vi "FrontPanel.vi"() -> ()   [LabVIEW 2017, in "WaveformGenerator.lvlib"]
uses:
  WaveformGenerator.lvlib
  WaveformSpecs.ctl
  WaveformGeneratorInterfaceRef.ctl
  <vilib>/DAQmx/write.llb/DAQmx Write (Analog 1D Wfm NChan NSamp).vi
  MessageQueue/QueueOperations/Enqueue Message (Single).vi
  FrontPanelReferences.vi
  <vilib>/DAQmx/miscellaneous.llb/DAQmx Fill In Error Info.vi
  MessageQueue/MessageQueue.lvlib
panel:
  in  "Field^2":dbl step=0.25
  in  "Waveform Specification":T1
  in  "Enum":enum16{"Initialize", "Idle", "Log", "Stop"}(ring)
  in  "Freq":dbl
  in  "Cone":bool
  in  "Radius":dbl step=0.025
  in  "Angle":dbl
  in  "stop":bool
  in  "OUT":bool caption="ON/OFF"
  out "Waveform Graph":waveform(dbl)[](graph)
  in  "Waveform Z":string(combo)="0" caption="Waveform"
  in  "Offset Z":dbl caption="Offset" min=-10.0 max=10.0 step=0.1
  in  "Phase Z":dbl caption="Phase" min=0.0 max=360.0 step=1.0
  in  "Amplitude Z":dbl caption="Amplitude" min=0.0 max=10.0 step=0.1
  in  "Frequency Z":dbl caption="Frequency" min=0.0 max=1000.0 step=0.1
  in  "Waveform Y":string(combo)="0" caption="Waveform"
  in  "Offset Y":dbl caption="Offset" min=-10.0 max=10.0 step=0.1
  in  "Phase Y":dbl caption="Phase" min=0.0 max=360.0 step=1.0
  in  "Amplitude Y":dbl caption="Amplitude" min=0.0 max=10.0 step=0.1
  in  "Frequency Y":dbl caption="Frequency" min=0.0 max=1000.0 step=0.1
  in  "Waveform X":string(combo)="0" caption="Waveform"
  in  "Offset X":dbl caption="Offset" min=-10.0 max=10.0 step=0.1
  in  "Phase X":dbl caption="Phase" min=0.0 max=360.0 step=1.0
  in  "Amplitude X":dbl caption="Amplitude" min=0.0 max=10.0 step=0.1
  in  "Frequency X":dbl caption="Frequency" min=0.0 max=1000.0 step=0.1
  # "Z Axis Coil"
  # "Y Axis Coil"
  # "X Axis Coil"
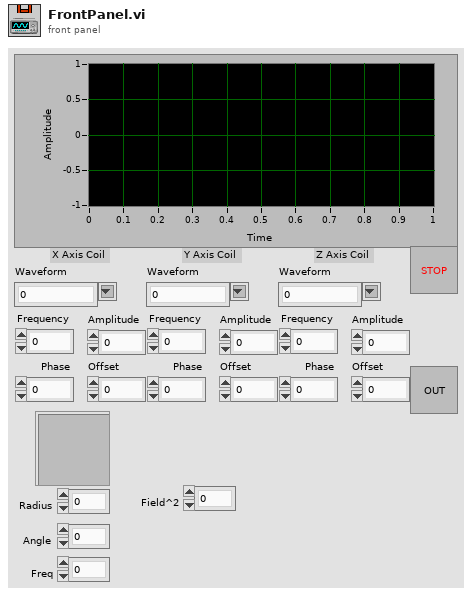
[diagram p1: front panel]
types:
  T1 = typedef "WaveformGenerator.lvlib/WaveformSpecs.ctl" = cluster{"X SignalType":enum16{"Sine Wave", "Triangle Wave", "Square Wave", "Sawtooth Wave"}, "X Offset":dbl, "X Frequency":dbl, "X Amplitude":dbl, "X Phase":dbl, "Y SignalType":enum16{"Sine Wave", "Triangle Wave", "Square Wave", "Sawtooth Wave"}, "Y Offset":dbl, "Y Frequency":dbl, "Y Amplitude":dbl, "Y Phase":dbl, "Z SignalType":enum16{"Sine Wave", "Triangle Wave", "Square Wave", "Sawtooth Wave"}, "Z Offset":dbl, "Z Frequency":dbl, "Z Amplitude":dbl, "Z Phase":dbl}
  T2 = typedef "WaveformGenerator.lvlib/WaveformGeneratorInterfaceRef.ctl" = cluster{"Waveform X":refnum<vi>, "Waveform Y":refnum<vi>, "Waveform Z":refnum<vi>, "Amplitude X":refnum<vi>, "Amplitude Y":refnum<vi>, "Amplitude Z":refnum<vi>, "Frequency X":refnum<vi>, "Frequency Y":refnum<vi>, "Frequency Z":refnum<vi>, "Phase X":refnum<vi>, "Phase Y":refnum<vi>, "Phase Z":refnum<vi>, "Offset X":refnum<vi>, "Offset Y":refnum<vi>, "Offset Z":refnum<vi>, "Stop":refnum<vi>, "On/Off":refnum<vi>, "Field^2":refnum<vi>}
  T3 = typedef "WaveformGenerator.lvlib/MessageQueue.lvlib/All Message Queues.ctl" = cluster{" Interface":refnum<queue>, "Log":refnum<queue>}
  T4 = cluster{"seconds since 1Jan1904":timestamp, "Waveform Specification":T1}
  T5 = enum16{"open", "replace", "create", "open or create", "replace or create", "replace or create with confirmation"}
  T6 = cluster{"Cone":bool, "Angle":dbl, "Radius":dbl, "Freq":dbl}
  T7 = cluster{"seconds since 1Jan1904":timestamp, "Waveform Specification out":T1}
  T8 = enum16{"Sine Wave", "Triangle Wave", "Square Wave", "Sawtooth Wave"}
  T9 = cluster{"Cone":bool, "Angle":dbl, dbl, "Freq":dbl}
  T10 = cluster{"Waveform Specification":T1, "NewVal":bool}
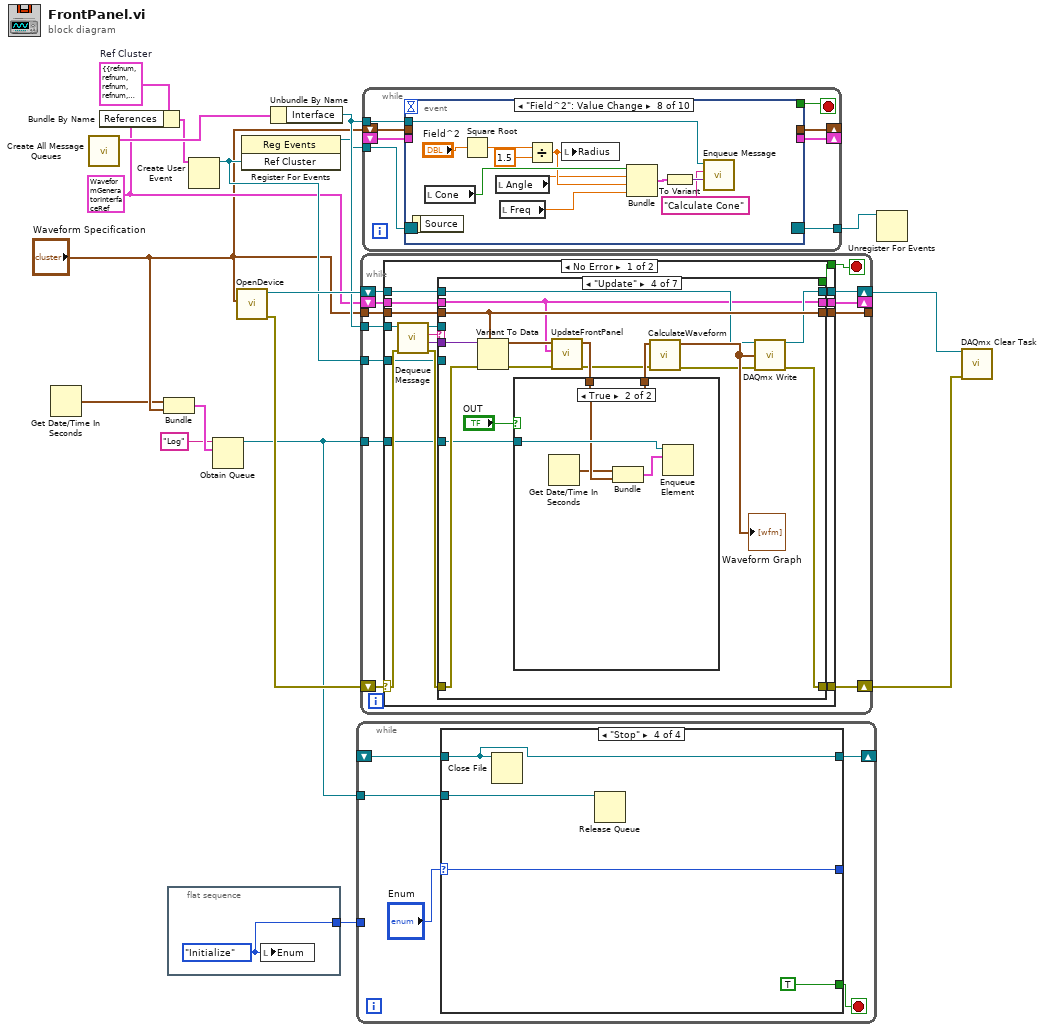
[diagram p0: block diagram]
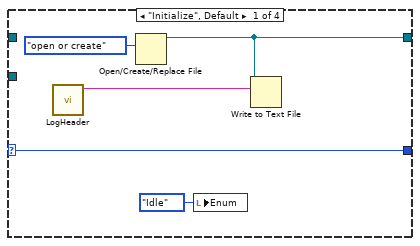
[diagram p2: hidden frame]
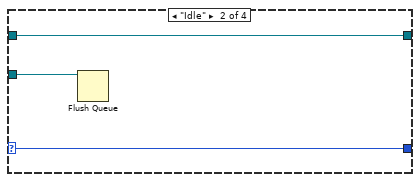
[diagram p3: hidden frame]
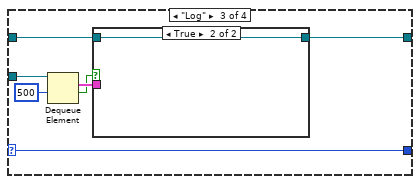
[diagram p4: hidden frame]
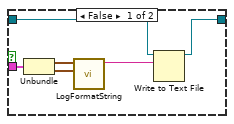
[diagram p5: hidden frame]
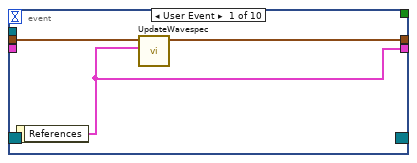
[diagram p6: hidden frame]
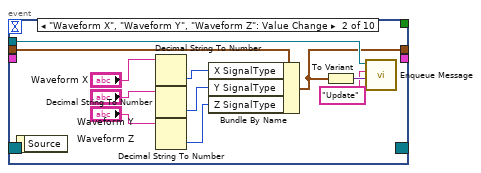
[diagram p7: hidden frame]
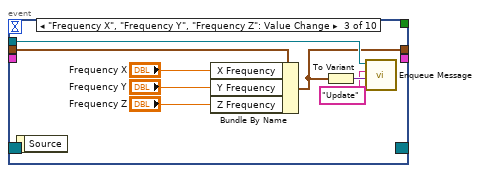
[diagram p8: hidden frame]
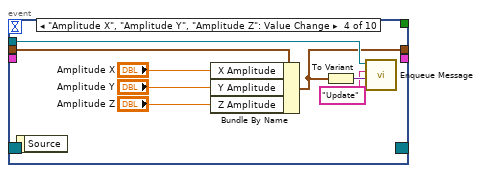
[diagram p9: hidden frame]
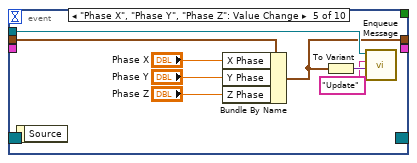
[diagram p10: hidden frame]
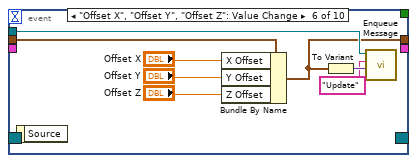
[diagram p11: hidden frame]
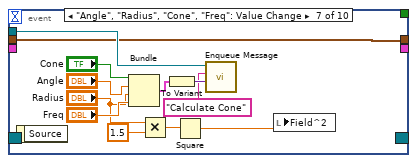
[diagram p12: hidden frame]
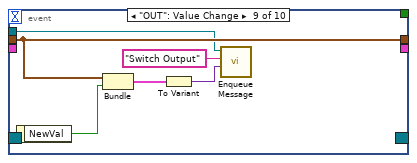
[diagram p13: hidden frame]
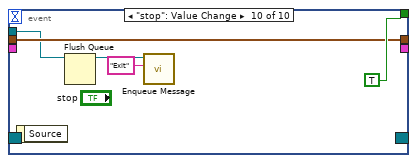
[diagram p14: hidden frame]
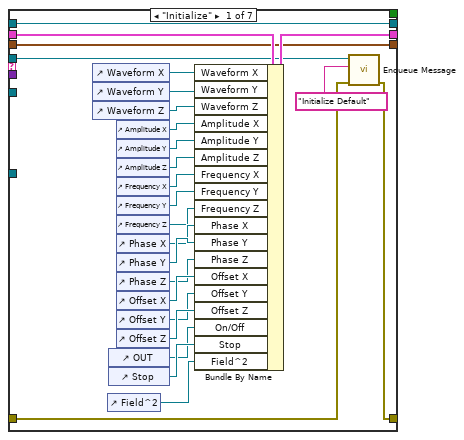
[diagram p15: hidden frame]
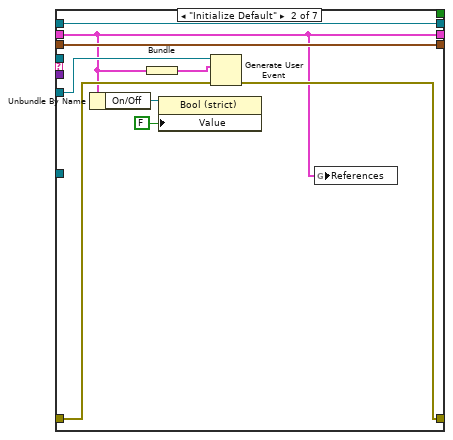
[diagram p16: hidden frame]
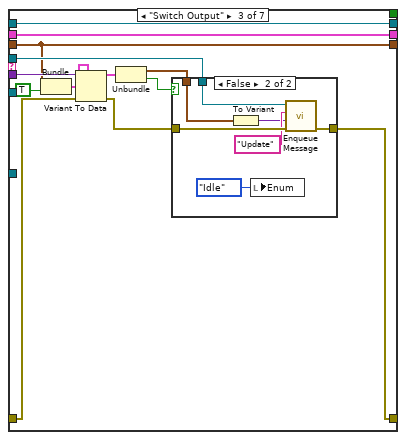
[diagram p17: hidden frame]
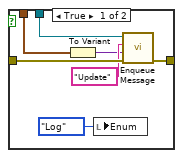
[diagram p18: hidden frame]
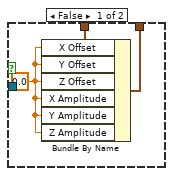
[diagram p19: hidden frame]
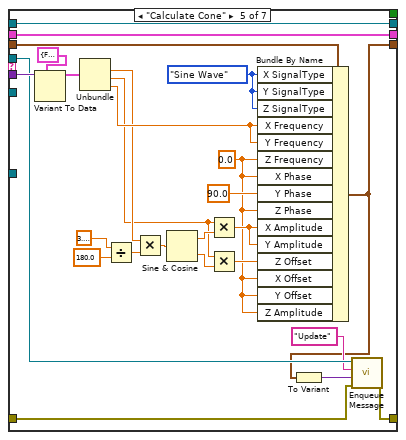
[diagram p20: hidden frame]
diagram:
  w9 = T2 {"Waveform X"=refnum, "Waveform Y"=refnum, "Waveform Z"=refnum, "Amplitude X"=refnum, "Amplitude Y"=refnum, "Amplitude Z"=refnum, "Frequency X"=refnum, "Frequency Y"=refnum, "Frequency Z"=refnum, "Phase X"=refnum, "Phase Y"=refnum, "Phase Z"=refnum, "Offset X"=refnum, "Offset Y"=refnum, "Offset Z"=refnum, "Stop"=refnum, "On/Off"=refnum, "Field^2"=refnum} ("Cluster")
  w7 = cluster{"References":T2} {"References"={"Waveform X"=refnum, "Waveform Y"=refnum, "Waveform Z"=refnum, "Amplitude X"=refnum, "Amplitude Y"=refnum, "Amplitude Z"=refnum, "Frequency X"=refnum, "Frequency Y"=refnum, "Frequency Z"=refnum, "Phase X"=refnum, "Phase Y"=refnum, "Phase Z"=refnum, "Offset X"=refnum, "Offset Y"=refnum, "Offset Z"=refnum, "Stop"=refnum, "On/Off"=refnum, "Field^2"=refnum}}  # Ref Cluster
  n1 = Get Date/Time In Seconds() -> (seconds since 1Jan1904=w1:timestamp)
  n2 = call "Create All Message Queues.vi"() -> ("Message Queues out"=w16:T3)  [unwired: 10 in, 1 out]
  n3 = Bundle By Name(cluster=w7, "References"=w9) -> (w8:cluster{"References":T2})
  n4 = Bundle("seconds since 1Jan1904"=w1, "Waveform Specification"="Waveform Specification") -> (w6:T4)  [unwired: 1 in]
  n5 = flat-sequence {
    tunnel: [w19] -> w3
    frame #0 {
      w19 = enum16{"Initialize", "Idle", "Log", "Stop"}."Initialize" ("Enum")
      n6 = local write "Enum"(w19) -> ()
    }
  }
  n7 = Create User Event(user event datatype=w8) -> (user event=w11:refnum<user-event>)  [unwired: 1 in, 1 out]
  n8 = Obtain Queue(name (unnamed)="Log", element data type=w6) -> (queue out=w4:refnum<queue>)  [unwired: 3 in, 2 out]
  n9 = call "OpenDevice.vi"("Waveform Specification"="Waveform Specification") -> ("error out"=w17:errorcluster, "Refnum out"=w18:refnum<k21>)  [unwired: 8 in, 1 out]
  n10 = register-events(w11) -> (reference out=w12:refnum<event-registration>)  [unwired: 2 in, 1 out]
  n11 = Unbundle By Name(w16) -> ("Interface"=w15:refnum<queue>)
  n12 = while {
    shift-right: [w24] -> _
    shift-left: _ -> [w23]
    tunnel: w4 -> [w22]
    tunnel: w3 -> [_]
    stop <- w21 stop-if-true
    n13 = case shown="\"Stop\"" "Enum" {
      selector: "Enum" -> [w29 w30 w35 w48]
      tunnel: [w25 w32 w36 w49] -> w24
      tunnel: w23 -> [_ w32 w37 w49]
      tunnel: w22 -> [_ w31 w39 w47]
      tunnel: [_ _ _ TRUE] -> w21
      tunnel: [w29 w30 w35 w48] -> _
      frame "Initialize", Default {
        n14 = call "LogHeader.vi"() -> ("String"=w26:string)  [unwired: 11 in]
        n15 = Open/Create/Replace File(operation (0:open)=T5."open or create") -> (refnum out=w25:refnum<file>)  [unwired: 5 in, 2 out]
        n16 = local write "Enum"(enum16{"Initialize", "Idle", "Log", "Stop"}."Idle" ("Enum")) -> ()
        n17 = Write to Text File(file (use dialog)=w25, text=w26) -> ()  [unwired: 2 in, 3 out]
      }
      frame "Idle" {
        n18 = Flush Queue(queue=w31) -> ()  [unwired: 1 in, 3 out]
      }
      frame "Log" {
        n19 = Dequeue Element(queue=w39, timeout in ms (-1)=500) -> (element=w38:T4, timed out?=w34:bool)  [unwired: 1 in, 2 out]
        n20 = case shown="True" w34 {
          tunnel: w38 -> [w45 _]
          tunnel: w37 -> [w41 w46]
          tunnel: [w40 w46] -> w36
          frame False {
            n21 = Unbundle(w45) -> ("seconds since 1Jan1904"=w43:timestamp, "Waveform Specification"=w44:T1)
            n22 = call "LogFormatString.vi"("Waveform Specification"=w44, "Timestamp"=w43) -> ("resulting string"=w42:string)  [unwired: 9 in]
            n23 = Write to Text File(file (use dialog)=w41, text=w42) -> (refnum out=w40:refnum<file>)  [unwired: 2 in, 2 out]
          }
          frame True {
          }
        }
      }
      frame "Stop" {
        n24 = Close File(refnum=w49) -> ()  [unwired: 1 in, 2 out]
        n25 = Release Queue(queue=w47) -> ()  [unwired: 2 in, 3 out]
      }
    }
  }
  n26 = while {
    tunnel: w15 -> [w62]
    shift-right: [w58] -> w14
    shift-left: w18 -> [w59]
    shift-right: [w60] -> w13
    shift-left: w17 -> [w61]
    shift-right: [w56] -> _
    shift-left: w9 -> [w57]
    tunnel: "Waveform Specification" -> [w55]
    tunnel: [w54] -> _
    tunnel: w11 -> [w52]
    tunnel: w4 -> [w51]
    stop <- w53 stop-if-true
    n27 = case shown="No Error" w61 {
      selector: w61 -> [w77 w206]
      tunnel: w62 -> [w78 _]
      tunnel: [w66 w204] -> w60
      tunnel: w59 -> [w73 w209]
      tunnel: [w68 w209] -> w58
      tunnel: w57 -> [w72 w208]
      tunnel: [w67 w208] -> w56
      tunnel: w55 -> [w71 w207]
      tunnel: [w70 w207] -> w54
      tunnel: [w69 _] -> w53
      tunnel: w52 -> [w64 _]
      tunnel: w51 -> [w63 _]
      frame No Error {
        n28 = call "Dequeue Message.vi"("error in (no error)"=w77, "Message Queue"=w78) -> ("error out"=w74:errorcluster, "Message Data"=w75:variant, "Message"=w76:string, "dup Message Queue"=w65:refnum<queue>)  [unwired: 6 in]
        n29 = case shown="\"Update\"" w76 {
          tunnel: w75 -> [_ _ w124 w155 w188 _ _]
          tunnel: w74 -> [w81 w108 w121 w150 w165 w192 w200]
          tunnel: w73 -> [w104 w113 w114 w152 w186 w198 w203]
          tunnel: w72 -> [w86 w105 w117 w142 w185 w195 w202]
          tunnel: w71 -> [w84 w109 w118 w156 w184 w196 w201]
          tunnel: [w84 w109 w118 w156 w166 w196 w201] -> w70
          tunnel: [_ _ _ _ _ TRUE _] -> w69
          tunnel: [w104 w113 w114 w151 w186 w197 w203] -> w68
          tunnel: [w85 w105 w117 w142 w185 w195 w202] -> w67
          tunnel: [w80 w107 w120 w148 w164 w194 w200] -> w66
          tunnel: w65 -> [w83 _ w119 _ w169 w193 _]
          tunnel: w64 -> [_ w110 _ _ _ _ _]
          tunnel: w63 -> [_ _ _ w141 _ _ _]
          frame "Initialize" {
            n30 = control-ref of="Waveform X"() -> (w87:refnum<vi>)
            n31 = control-ref of="Waveform Y"() -> (w88:refnum<vi>)
            n32 = control-ref of="Waveform Z"() -> (w89:refnum<vi>)
            n33 = control-ref of="Field^2"() -> (w79:refnum<vi>)
            n34 = control-ref of="OUT"() -> (w102:refnum<vi>)
            n35 = control-ref of="Stop"() -> (w103:refnum<vi>)
            n36 = control-ref of="Amplitude X"() -> (w90:refnum<vi>)
            n37 = control-ref of="Amplitude Y"() -> (w91:refnum<vi>)
            n38 = control-ref of="Amplitude Z"() -> (w92:refnum<vi>)
            n39 = control-ref of="Frequency X"() -> (w93:refnum<vi>)
            n40 = control-ref of="Frequency Y"() -> (w94:refnum<vi>)
            n41 = control-ref of="Frequency Z"() -> (w95:refnum<vi>)
            n42 = control-ref of="Phase X"() -> (w96:refnum<vi>)
            n43 = control-ref of="Phase Y"() -> (w97:refnum<vi>)
            n44 = control-ref of="Phase Z"() -> (w98:refnum<vi>)
            n45 = control-ref of="Offset X"() -> (w99:refnum<vi>)
            n46 = control-ref of="Offset Y"() -> (w100:refnum<vi>)
            n47 = control-ref of="Offset Z"() -> (w101:refnum<vi>)
            n48 = Bundle By Name(cluster=w86, "Waveform X"=w87, "Waveform Y"=w88, "Waveform Z"=w89, "Amplitude X"=w90, "Amplitude Y"=w91, "Amplitude Z"=w92, "Frequency X"=w93, "Frequency Y"=w94, "Frequency Z"=w95, "Phase X"=w96, "Phase Y"=w97, "Phase Z"=w98, "Offset X"=w99, "Offset Y"=w100, "Offset Z"=w101, "On/Off"=w102, "Stop"=w103, "Field^2"=w79) -> (w85:T2)
            n49 = call-poly "Enqueue Message.vi"("error in (no error)"=w81, "Message"="Initialize Default", "Message Queue"=w83) -> ("error out"=w80:errorcluster)  [unwired: 7 in, 1 out]
          }
          frame "Initialize Default" {
            n50 = Unbundle By Name(w105) -> ("On/Off"=w112:refnum<vi>)
            n51 = Bundle("Cluster"=w105) -> (w106:cluster{"Cluster":T2})  [unwired: 1 in]
            n52 = property class="Bool (strict)"(reference=w112, "Value"=FALSE) -> ()  [unwired: 1 in, 2 out]
            n53 = Generate User Event(user event=w110, event data cluster=w106, error in=w108) -> (error out=w107:errorcluster)  [unwired: 1 in, 1 out]
            n54 = global write "FrontPanelReferences.vi" "References"(w105) -> ()
          }
          frame "Switch Output" {
            n55 = Bundle("Waveform Specification"=w118, TRUE) -> (w125:cluster{"Waveform Specification":T1, bool})  [unwired: 1 in]
            n56 = Variant To Data(error in=w121, type=w125, Variant=w124) -> (data=w123:cluster{"Waveform Specification":T1, bool}, error out=w122:errorcluster)
            n57 = Unbundle(w123) -> ("Waveform Specification"=w115:T1, w116:bool)
            n58 = case shown="False" w116 {
              tunnel: w122 -> [w132 w139]
              tunnel: [w131 w138] -> w120
              tunnel: w119 -> [w133 w140]
              tunnel: w115 -> [w128 w135]
              frame True {
                n59 = To Variant(anything=w128) -> (Variant=w129:variant)
                n60 = local write "Enum"(enum16{"Initialize", "Idle", "Log", "Stop"}."Log" ("Enum")) -> ()
                n61 = call-poly "Enqueue Message.vi"("error in (no error)"=w132, "Message Data"=w129, "Message"="Update", "Message Queue"=w133) -> ("error out"=w131:errorcluster)  [unwired: 6 in, 1 out]
              }
              frame False {
                n62 = To Variant(anything=w135) -> (Variant=w136:variant)
                n63 = local write "Enum"(enum16{"Initialize", "Idle", "Log", "Stop"}."Idle" ("Enum")) -> ()
                n64 = call-poly "Enqueue Message.vi"("error in (no error)"=w139, "Message Data"=w136, "Message"="Update", "Message Queue"=w140) -> ("error out"=w138:errorcluster)  [unwired: 6 in, 1 out]
              }
            }
          }
          frame "Update" {
            n65 = Variant To Data(error in=w150, type=w156, Variant=w155) -> (data=w145:T1, error out=w144:errorcluster)
            n66 = call "UpdateFrontPanel.vi"("error in"=w144, "Cluster"=w142, "Waveform Specification in"=w145) -> ("error out"=w143:errorcluster, "Waveform Specification out"=w146:T1)  [unwired: 7 in]
            n67 = case shown="True" "OUT" {
              tunnel: w146 -> [w159 w161]
              tunnel: [w157 w161] -> w154
              tunnel: w141 -> [_ w163]
              frame False {
                w158 = 0.0 ("Y Offset")
                n68 = Bundle By Name(cluster=w159, "X Offset"=w158, "Y Offset"=w158, "Z Offset"=w158, "X Amplitude"=w158, "Y Amplitude"=w158, "Z Amplitude"=w158) -> (w157:T1)
              }
              frame True {
                n69 = Get Date/Time In Seconds() -> (seconds since 1Jan1904=w160:timestamp)
                n70 = Bundle("seconds since 1Jan1904"=w160, "Waveform Specification out"=w161) -> (w162:T7)  [unwired: 1 in]
                n71 = Enqueue Element(queue=w163, element=w162) -> ()  [unwired: 2 in, 3 out]
              }
            }
            n72 = call "CalculateWaveform.vi"("error out"=w143, "Waveform Specification"=w154) -> ("error in"=w149:errorcluster, "Array"=w153:waveform(dbl)[])  [unwired: 8 in]
            "Waveform Graph" <- w153
            n73 = call-poly <vilib>:"DAQmx Write.vi"("task/channels in"=w152, "data"=w153, "error in"=w149) -> ("task out"=w151:refnum<k21>, "error out"=w148:errorcluster)  [unwired: 10 in, 1 out]
          }
          frame "Calculate Cone" {
            w170 = 0.0 ("Z Frequency")
            w183 = T8."Sine Wave" ("X Signal Type")
            n74 = Variant To Data(type=T6 {"Cone"=FALSE, "Angle"=0.0, "Radius"=0.0, "Freq"=0.0}, Variant=w188) -> (data=w187:T6)  [unwired: 1 in, 1 out]
            n75 = Unbundle(w187) -> ("Angle"=w176:dbl, "Radius"=w172:dbl, "Freq"=w182:dbl)  [unwired: 1 out]
            n76 = Divide(x=3.141592653589793, y=180.0) -> (x/y=w178:dbl)
            n77 = Multiply(x=w176, y=w178) -> (x*y=w177:dbl)
            n78 = Sine & Cosine(0:w177) -> (1:w175:dbl, 2:w173:dbl)
            n79 = Multiply(x=w172, y=w175) -> (x*y=w174:dbl)
            n80 = Multiply(x=w172, y=w173) -> (x*y=w171:dbl)
            n81 = Bundle By Name(cluster=w184, "X SignalType"=w183, "Y SignalType"=w183, "Z SignalType"=w183, "X Frequency"=w182, "Y Frequency"=w182, "Z Frequency"=w170, "X Phase"=w170, "Y Phase"=90.0, "Z Phase"=w170, "X Amplitude"=w174, "Y Amplitude"=w174, "Z Offset"=w171, "X Offset"=w170, "Y Offset"=w170, "Z Amplitude"=w170) -> (w166:T1)
            n82 = To Variant(anything=w166) -> (Variant=w167:variant)
            n83 = call-poly "Enqueue Message.vi"("error in (no error)"=w165, "Message Data"=w167, "Message"="Update", "Message Queue"=w169) -> ("error out"=w164:errorcluster)  [unwired: 6 in, 1 out]
          }
          frame "Exit" {
            n84 = Release Queue(queue=w193, error in (no error)=w192) -> (error out=w191:errorcluster)  [unwired: 1 in, 2 out]
            n85 = call <vilib>:"DAQmx Stop Task.vi"("task/channels in"=w198, "error in"=w191) -> ("task out"=w197:refnum<k21>, "error out"=w194:errorcluster)  [unwired: 12 in]
            n86 = local write "Enum"(enum16{"Initialize", "Idle", "Log", "Stop"}."Stop" ("Enum")) -> ()
          }
          frame Default {
          }
        }
      }
      frame Error {
        n87 = call <vilib>:"Simple Error Handler.vi"("error in (no error)"=w206) -> ("error out"=w205:errorcluster)  [unwired: 4 in, 4 out]
        n88 = call <vilib>:"Clear Errors.vi"("error in (no error)"=w205) -> ("error out"=w204:errorcluster)  [unwired: 5 in, 1 out]
      }
    }
  }
  n89 = while {
    tunnel: w15 -> [w217]
    shift-right: [w215] -> _
    shift-left: "Waveform Specification" -> [w216]
    tunnel: w12 -> [w213]
    tunnel: [w212] -> w10
    shift-right: [w211] -> _
    shift-left: _ -> [w210]
    stop <- w214 stop-if-true
    n90 = event shown="[7] \"Field^2\": Value Change" {
      selector: w213 -> [_ _ _ _ _ _ _ _ _ _]
      dyn-events: [_ _ _ _ _ _ _ _ _ _] -> w212
      timeout: _ -> [_ _ _ _ _ _ _ _ _ _]
      tunnel: w217 -> [_ w230 w238 w246 w254 w262 w274 w280 w287 w294]
      tunnel: w216 -> [w220 w228 w236 w244 w252 w260 w271 _ w288 w296]
      tunnel: [w219 w227 w235 w243 w251 w259 w271 _ w288 w296] -> w215
      tunnel: [_ _ _ _ _ _ _ _ _ TRUE] -> w214
      tunnel: [w218 _ _ _ _ _ _ _ _ _] -> w211
      tunnel: w210 -> [_ _ _ _ _ _ _ _ _ _]
      event User Event {
        n91 = event-data() -> ("References"=w218:T2)  [unwired: 1 in]
        n92 = call "UpdateWavespec.vi"("Cluster"=w218, "Waveform Specification in"=w220) -> ("Waveform Specification out"=w219:T1)  [unwired: 8 in, 1 out]
      }
      event "Waveform X", "Waveform Y", "Waveform Z": Value Change {
        n93 = event-data() -> ()  [unwired: 1 in, 1 out]
        n94 = Decimal String To Number(string="Waveform X") -> (number=w224:i32)  [unwired: 2 in, 1 out]
        n95 = Decimal String To Number(string="Waveform Y") -> (number=w225:i32)  [unwired: 2 in, 1 out]
        n96 = Decimal String To Number(string="Waveform Z") -> (number=w226:i32)  [unwired: 2 in, 1 out]
        n97 = Bundle By Name(cluster=w228, "X SignalType"=w224, "Y SignalType"=w225, "Z SignalType"=w226) -> (w227:T1)
        n98 = To Variant(anything=w227) -> (Variant=w231:variant)
        n99 = call-poly "Enqueue Message.vi"("Message Data"=w231, "Message"="Update", "Message Queue"=w230) -> ()  [unwired: 7 in, 2 out]
      }
      event "Frequency X", "Frequency Y", "Frequency Z": Value Change {
        n100 = event-data() -> ()  [unwired: 1 in, 1 out]
        n101 = Bundle By Name(cluster=w236, "X Frequency"="Frequency X", "Y Frequency"="Frequency Y", "Z Frequency"="Frequency Z") -> (w235:T1)
        n102 = To Variant(anything=w235) -> (Variant=w239:variant)
        n103 = call-poly "Enqueue Message.vi"("Message Data"=w239, "Message"="Update", "Message Queue"=w238) -> ()  [unwired: 7 in, 2 out]
      }
      event "Amplitude X", "Amplitude Y", "Amplitude Z": Value Change {
        n104 = event-data() -> ()  [unwired: 1 in, 1 out]
        n105 = Bundle By Name(cluster=w244, "X Amplitude"="Amplitude X", "Y Amplitude"="Amplitude Y", "Z Amplitude"="Amplitude Z") -> (w243:T1)
        n106 = To Variant(anything=w243) -> (Variant=w247:variant)
        n107 = call-poly "Enqueue Message.vi"("Message Data"=w247, "Message"="Update", "Message Queue"=w246) -> ()  [unwired: 7 in, 2 out]
      }
      event "Phase X", "Phase Y", "Phase Z": Value Change {
        n108 = event-data() -> ()  [unwired: 1 in, 1 out]
        n109 = Bundle By Name(cluster=w252, "X Phase"="Phase X", "Y Phase"="Phase Y", "Z Phase"="Phase Z") -> (w251:T1)
        n110 = To Variant(anything=w251) -> (Variant=w255:variant)
        n111 = call-poly "Enqueue Message.vi"("Message Data"=w255, "Message"="Update", "Message Queue"=w254) -> ()  [unwired: 7 in, 2 out]
      }
      event "Offset X", "Offset Y", "Offset Z": Value Change {
        n112 = event-data() -> ()  [unwired: 1 in, 1 out]
        n113 = Bundle By Name(cluster=w260, "X Offset"="Offset X", "Y Offset"="Offset Y", "Z Offset"="Offset Z") -> (w259:T1)
        n114 = To Variant(anything=w259) -> (Variant=w263:variant)
        n115 = call-poly "Enqueue Message.vi"("Message Data"=w263, "Message"="Update", "Message Queue"=w262) -> ()  [unwired: 7 in, 2 out]
      }
      event "Angle", "Radius", "Cone", "Freq": Value Change {
        n116 = event-data() -> ()  [unwired: 1 in, 1 out]
        n117 = Bundle("Cone"="Cone", "Angle"="Angle", "Radius"="Radius", "Freq"="Freq") -> (w270:T6)  [unwired: 1 in]
        n118 = Multiply(x="Radius", y=1.5) -> (x*y=w265:dbl)
        n119 = To Variant(anything=w270) -> (Variant=w269:variant)
        n120 = Square(x=w265) -> (x^2=w264:dbl)
        n121 = call-poly "Enqueue Message.vi"("Message Data"=w269, "Message"="Calculate Cone", "Message Queue"=w274) -> ()  [unwired: 7 in, 2 out]
        n122 = local write "Field^2"(w264) -> ()
      }
      event "Field^2": Value Change {
        n123 = event-data() -> ()  [unwired: 1 in, 1 out]
        n124 = local read "Cone"() -> (w279:bool)
        n125 = Square Root(x="Field^2") -> (sqrt(x)=w285:dbl)
        n126 = local read "Angle"() -> (w277:dbl)
        n127 = local read "Freq"() -> (w276:dbl)
        n128 = Divide(x=w285, y=1.5) -> (x/y=w278:dbl)
        n129 = local write "Radius"(w278) -> ()
        n130 = Bundle("Cone"=w279, "Angle"=w277, w278, "Freq"=w276) -> (w283:T9)  [unwired: 1 in]
        n131 = To Variant(anything=w283) -> (Variant=w282:variant)
        n132 = call-poly "Enqueue Message.vi"("Message Data"=w282, "Message"="Calculate Cone", "Message Queue"=w280) -> ()  [unwired: 7 in, 2 out]
      }
      event "OUT": Value Change {
        n133 = event-data() -> ("NewVal"=w291:bool)  [unwired: 1 in]
        n134 = Bundle("Waveform Specification"=w288, "NewVal"=w291) -> (w290:T10)  [unwired: 1 in]
        n135 = To Variant(anything=w290) -> (Variant=w289:variant)
        n136 = call-poly "Enqueue Message.vi"("Message Data"=w289, "Message"="Switch Output", "Message Queue"=w287) -> ()  [unwired: 7 in, 2 out]
      }
      event "stop": Value Change {
        n137 = event-data() -> ()  [unwired: 1 in, 1 out]
        n138 = Flush Queue(queue=w294) -> (queue out=w293:refnum<queue>)  [unwired: 1 in, 2 out]
        n139 = call-poly "Enqueue Message.vi"("Message"="Exit", "Message Queue"=w293) -> ()  [unwired: 8 in, 2 out]
      }
    }
  }
  n140 = Unregister For Events(event registration refnum=w10) -> ()  [unwired: 1 in, 1 out]
  n141 = call <vilib>:"DAQmx Clear Task.vi"("task in"=w14, "error in"=w13) -> ()  [unwired: 13 in, 1 out]
